vi "mecanum_tank_1_sl.vi"   [LabVIEW 2012, in "Mecanum Drive.lvrbt"]
uses:
  Mecanum Drive.lvrbt
  <vilib>/NXT/Hardware/Plugins/Tetrix DC Motor/TetrixDCMotorAddress.ctl
  <vilib>/NXT/Dual Mode Library/Display/drawNumber.vi
  <vilib>/NXT/NXTIO Xnodes/NXTIONodeSubVIs/TETRIX IO Move DC Motors.vi
  <vilib>/NXT/NXTIO Xnodes/NXTIONodeSubVIs/TETRIX IO Check Battery.vi
  <vilib>/NXT/NXTIO Xnodes/NXTIONodeSubVIs/TETRIX IO Stop DC Motors.vi
  <vilib>/NXT/NXTIO Xnodes/AddressXNode/NXTIOAddress.xnode
  <vilib>/NXT/Subs/LVHSConnector.ctl
  <vilib>/NXT/NXTIO Xnodes/NXTIOXNode/NXTIO.xnode
  <vilib>/NXT/LegoClasses/BrickReference/BrickReference.lvclass
panel:
  # "This VI was generated based on your configuration in the Remote Control Editor. You may modify the code as needed for your robot. To test this program for an FTC match, return to the Remote Control Editor, select the \"Run Program\" tab, and choose \"Teleop\"."
types:
  T1 = typedef "TetrixDCMotorAddress.ctl" = i32
  T2 = cluster{"TetrixDCMotor":T1, "TetrixDCMotor 2":T1}
  T3 = typedef "LVHSConnector.ctl" = refnum<class "BrickReference.lvclass">
  T4 = typedef "FTC ControllerState.ctl" = cluster{"Left X":i8, "Left Y":i8, "Right X":i8, "Right Y":i8, "Button Encoding 9-12":u8, "Button Encoding 1-8":u8, "POV":T5}
  T5 = typedef "FTC POVState.ctl" = i8
  T6 = typedef "FTC ButtonEventType.ctl" = enum16{"Pressed", "Released"}
  T7 = cluster{"Button ID":enum16{"None", "Button 1", "Button 2", "Button 3", "Button 4", "Button 5", "Button 6", "Button 7", "Button 8", "Button 9", "Button 10", "Button 11", "Button 12", "POV Up", "POV Up Right", "POV Right", "POV Down Right", "POV Down", "POV Down Left", "POV Left", "POV Up Left"}, "Event Type":T6}[]
  T8 = typedef "FTC ButtonState.ctl" = cluster{"Button 1":bool, "Button 2":bool, "Button 3":bool, "Button 4":bool, "Button 5":bool, "Button 6":bool, "Button 7":bool, "Button 8":bool, "Button 9":bool, "Button 10":bool, "Button 11":bool, "Button 12":bool, "POV":T5}
  T9 = enum16{"None", "Button 1", "Button 2", "Button 3", "Button 4", "Button 5", "Button 6", "Button 7", "Button 8", "Button 9", "Button 10", "Button 11", "Button 12", "POV Up", "POV Up Right", "POV Right", "POV Down Right", "POV Down", "POV Down Left", "POV Left", "POV Up Left"}
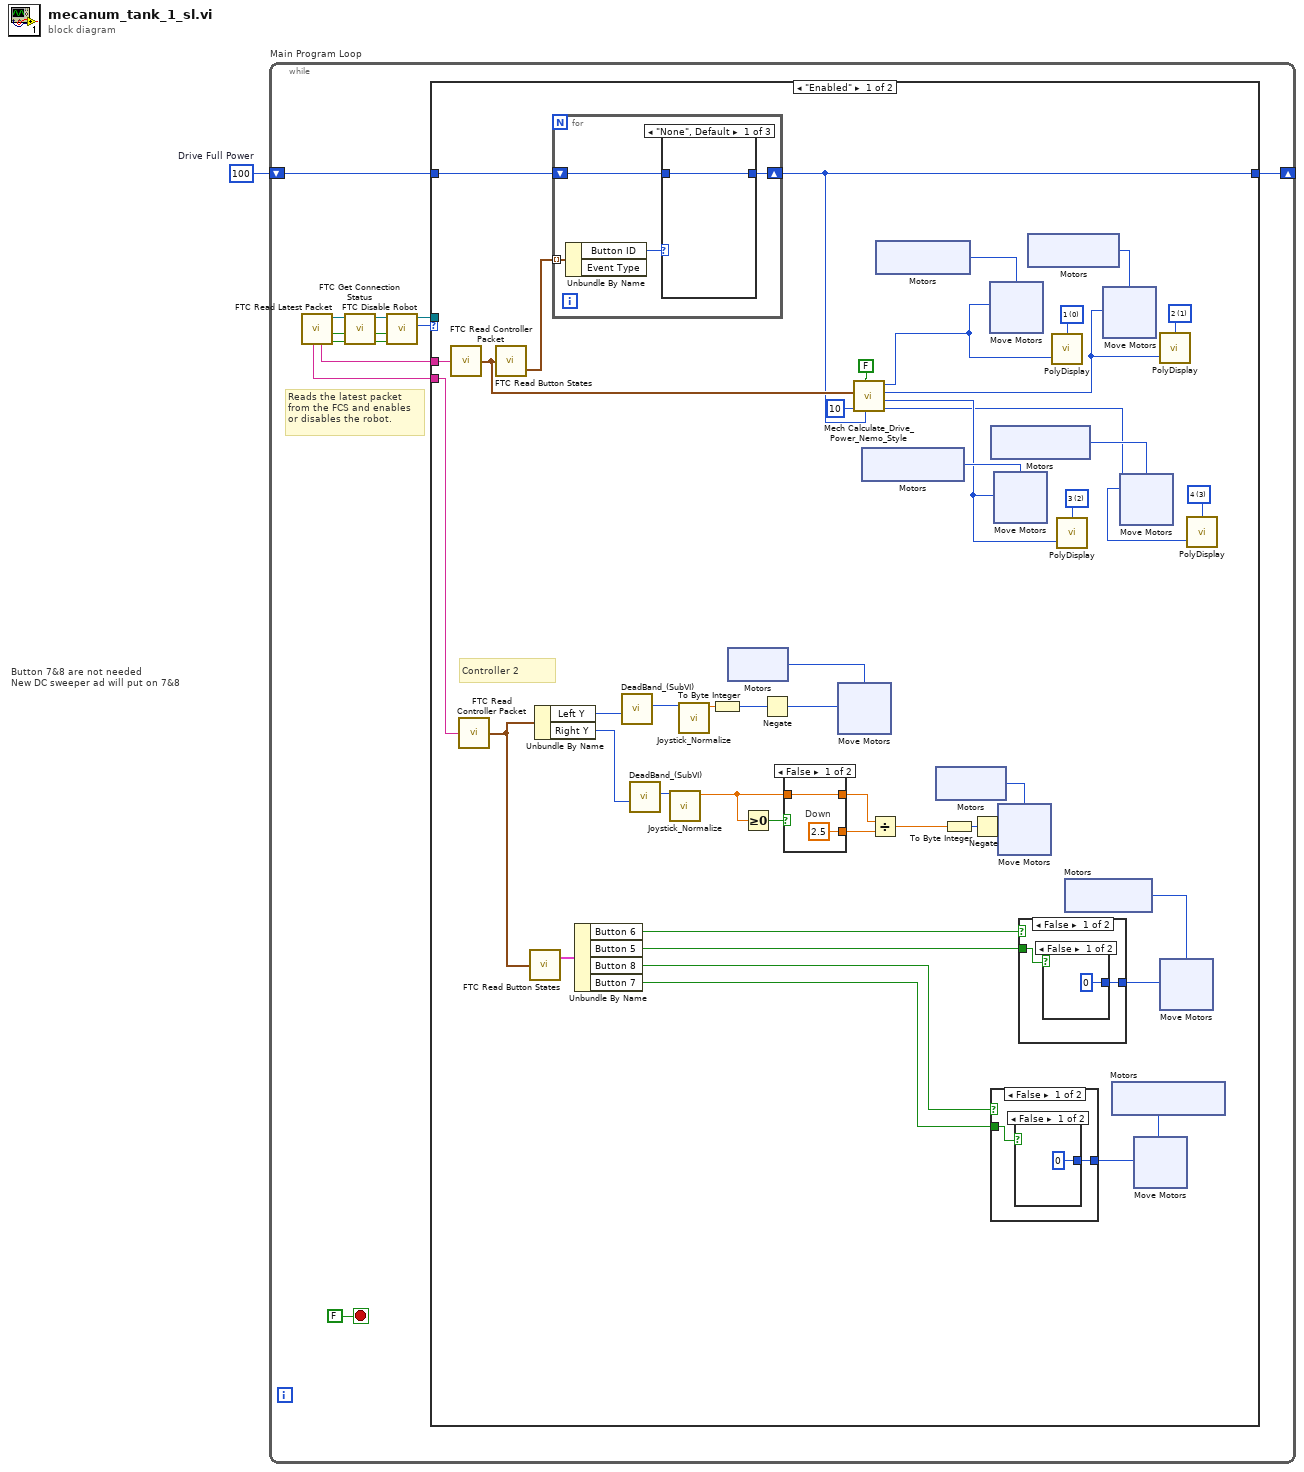
[diagram p0: block diagram]
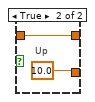
[diagram p2: hidden frame]
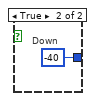
[diagram p3: hidden frame]
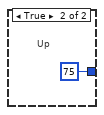
[diagram p4: hidden frame]
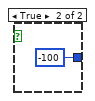
[diagram p5: hidden frame]
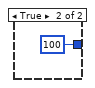
[diagram p6: hidden frame]
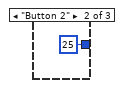
[diagram p7: hidden frame]
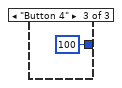
[diagram p8: hidden frame]
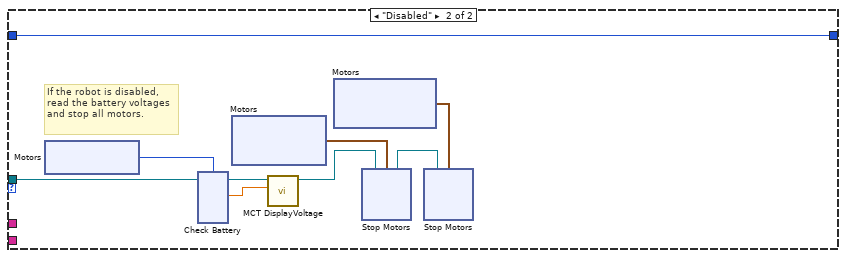
[diagram p9: hidden frame]
diagram:
  w1 = 100  # Drive Full Power
  # "Button 7&8 are not needed\nNew DC sweeper ad will put on 7&8"
  n1 = while "Main Program Loop" {
    shift-right: [w2] -> _
    shift-left: w1 -> [w3]
    stop <- FALSE stop-if-true
    # "Reads the latest packet\nfrom the FCS and enables\nor disables the robot."
    n2 = call <vilib>:"FTC Read Latest Packet.vi"() -> ("Packet Received?"=w11:bool, "Stopped?"=w8:bool, "NXT"=w10:T3, "Controller 1"=w13:string, "Controller 2"=w12:string)  [unwired: 6 in, 1 out]
    n3 = call <vilib>:"FTC Get Connection Status.vi"("Packet Received?"=w11, "Stopped?"=w8, "NXT"=w10) -> ("Online?"=w5:bool, "Stopped?"=w6:bool, "NXT"=w7:T3)  [unwired: 5 in]
    n4 = call <vilib>:"FTC Disable Robot.vi"("Online?"=w5, "Stopped?"=w6, "NXT"=w7) -> ("Enabled?"=w9:enum16{"Disabled", "Enabled"}, "NXT"=w4:T3)  [unwired: 3 in]
    n5 = case "disableCase" shown="\"Enabled\"" w9 {
      tunnel: w13 -> [w60 _]
      tunnel: w12 -> [w59 _]
      tunnel: w4 -> [_ w154]
      tunnel: w3 -> [w56 w146]
      tunnel: [w55 w146] -> w2
      frame "Enabled" {
        w21 = i16 3 items=["1", "2", "3", "4", "5", "6", "7", "8", "9", "10", "11", "12"] ("Line")
        w23 = i16 2 items=["1", "2", "3", "4", "5", "6", "7", "8", "9", "10", "11", "12"] ("Line")
        w25 = i16 1 items=["1", "2", "3", "4", "5", "6", "7", "8", "9", "10", "11", "12"] ("Line")
        w26 = i16 0 items=["1", "2", "3", "4", "5", "6", "7", "8", "9", "10", "11", "12"] ("Line")
        # "Controller 2"
        n6 = call <vilib>:"FTC Read Controller Packet.vi"("Packet"=w60) -> ("Controller State"=w57:T4)  [unwired: 4 in]
        n7 = call <vilib>:"FTC Read Controller Packet.vi"("Packet"=w59) -> ("Controller State"=w48:T4)  [unwired: 4 in]
        n8 = call <vilib>:"FTC Read Button States.vi"("Controller State"=w57) -> ("Button Events"=w58:T7)  [unwired: 2 in, 1 out]
        n9 = call <vilib>:"FTC Read Button States.vi"("Controller State"=w48) -> ("Button States"=w47:T8)  [unwired: 2 in, 1 out]
        n10 = Unbundle By Name(w48) -> ("Left Y"=w54:i8, "Right Y"=w49:i8)
        n11 = for {
          tunnel: w58 -> [w142] mode=indexing
          shift-right: [w140] -> w55
          shift-left: w56 -> [w139]
          n12 = Unbundle By Name(w142) -> ("Button ID"=w141:T9)  [unwired: 1 out]
          n13 = case shown="\"None\", Default" w141 {
            tunnel: [w143 25 100] -> w140
            tunnel: w139 -> [w143 _ _]
            frame "None", Default {
            }
            frame "Button 2" {
            }
            frame "Button 4" {
            }
          }
        }
        n14 = Unbundle By Name(w47) -> ("Button 6"=w44:bool, "Button 5"=w43:bool, "Button 8"=w39:bool, "Button 7"=w38:bool)
        n15 = call "DeadBand_(SubVI).vi"("Axis In"=w54) -> ("Axis out"=w53:i8)  [unwired: 10 in]
        n16 = call "DeadBand_(SubVI).vi"("Axis In"=w49) -> ("Axis out"=w50:i8)  [unwired: 10 in]
        n17 = call "Joystick_Normalize.vi"("Joystick In"=w50) -> ("Norm Out"=w33:sgl)  [unwired: 10 in]
        n18 = call "Joystick_Normalize.vi"("Joystick In"=w53) -> ("Norm Out"=w52:sgl)  [unwired: 10 in]
        n19 = To Byte Integer(number=w52) -> (8bit integer=w35:i8)
        n20 = xnode "Motors"() -> ("Motor"=w51:T1)
        n21 = Greater Or Equal To 0?(x=w33) -> (x >= 0?=w17:bool)
        n22 = Negate(x=w35) -> (-x=w34:i8)
        n23 = case shown="False" w17 {
          tunnel: [w62 w64] -> w15
          tunnel: w33 -> [w62 w64]
          tunnel: [sgl 2.5 sgl 10.0] -> w16
          frame False {
            # "Down"
          }
          frame True {
            # "Up"
          }
        }
        n24 = xnode "Move Motors"("Power/Speed 1"=w34, "Motors"=w51) -> ()  [unwired: 1 in, 1 out]
        n25 = call "Mech Calculate_Drive_Power_Nemo_Style.vi"("Power"=w55, "Reverse"=FALSE, "Deadband (10)"=i8 10, "Controller State"=w57) -> ("Right Rear Power"=w20:i8, "Right Front Power"=w22:i8, "Left Rear Power"=w24:i8, "Left Front Power"=w19:i8)  [unwired: 4 in]
        n26 = xnode ("Motors")() -> ("Motor"=w31:T1)
        n27 = Divide(x=w15, y=w16) -> (x/y=w36:sgl)
        n28 = xnode ("Motors")() -> ("Motor"=w28:T1)
        n29 = xnode "Motors"() -> ("Motor"=w46:T1)
        n30 = To Byte Integer(number=w36) -> (8bit integer=w45:i8)
        n31 = Negate(x=w45) -> (-x=w37:i8)
        n32 = xnode ("Move Motors")("Power/Speed 1"=w19, "Motors"=w28) -> ()  [unwired: 1 in, 1 out]
        n33 = xnode ("Motors")() -> ("Motor"=w30:T1)
        n34 = case shown="False" w39 {
          tunnel: w38 -> [w105 _]
          tunnel: [w104 i8 75] -> w32
          frame False {
            n35 = case shown="False" w105 {
              tunnel: [i8 0 i8 -40] -> w104
              frame False {
              }
              frame True {
                # "Down"
              }
            }
          }
          frame True {
            # "Up"
          }
        }
        n36 = xnode ("Move Motors")("Power/Speed 1"=w22, "Motors"=w31) -> ()  [unwired: 1 in, 1 out]
        n37 = xnode "Move Motors"("Power/Speed 1"=w37, "Motors"=w46) -> ()  [unwired: 1 in, 1 out]
        n38 = case shown="False" w44 {
          tunnel: w43 -> [w119 _]
          tunnel: [w118 i8 100] -> w41
          frame False {
            n39 = case shown="False" w119 {
              tunnel: [i8 0 i8 -100] -> w118
              frame False {
              }
              frame True {
              }
            }
          }
          frame True {
          }
        }
        n40 = xnode ("Motors")() -> ("Motor"=w29:T1)
        n41 = call-poly <vilib>:"PolyDisplay.vi"("number"=w19, "Line"=w26) -> ()  [unwired: 2 in, 1 out]
        n42 = call-poly <vilib>:"PolyDisplay.vi"("number"=w22, "Line"=w23) -> ()  [unwired: 2 in, 1 out]
        n43 = xnode "Motors"() -> ("Motor"=w42:T1)
        n44 = xnode ("Move Motors")("Power/Speed 1"=w24, "Motors"=w29) -> ()  [unwired: 1 in, 1 out]
        n45 = xnode "Motors"() -> ("Motor"=w40:T1)
        n46 = xnode ("Move Motors")("Power/Speed 1"=w20, "Motors"=w30) -> ()  [unwired: 1 in, 1 out]
        n47 = xnode "Move Motors"("Power/Speed 1"=w32, "Motors"=w40) -> ()  [unwired: 1 in, 1 out]
        n48 = call-poly <vilib>:"PolyDisplay.vi"("number"=w24, "Line"=w25) -> ()  [unwired: 2 in, 1 out]
        n49 = xnode "Move Motors"("Power/Speed 1"=w41, "Motors"=w42) -> ()  [unwired: 1 in, 1 out]
        n50 = call-poly <vilib>:"PolyDisplay.vi"("number"=w20, "Line"=w21) -> ()  [unwired: 2 in, 1 out]
      }
      frame "Disabled" {
        # "If the robot is disabled, read the battery voltages and stop all motors."
        n51 = xnode ("Motors")() -> ("Motor"=w153:T1)
        n52 = xnode ("Check Battery")("Motors"=w153, "NXT/EV3"=w154) -> ("Voltage 1"=w152:sgl, "NXT/EV3"=w151:T3)
        n53 = xnode "Motors"() -> ("Motor"=w150:cluster{"TetrixDCMotor":T1, "TetrixDCMotor":T1})
        n54 = call <vilib>:"MCT DisplayVoltage.vi"("Motor Voltage"=w152, "NXT"=w151) -> ("NXT"=w149:T3)  [unwired: 9 in]
        n55 = xnode "Motors"() -> ("Motor"=w148:cluster{"TetrixDCMotor":T1, "TetrixDCMotor":T1})
        n56 = xnode "Stop Motors"("Motors"=w150, "NXT/EV3"=w149) -> ("NXT/EV3"=w147:T3)
        n57 = xnode "Stop Motors"("Motors"=w148, "NXT/EV3"=w147) -> ()  [unwired: 1 out]
      }
    }
  }
